vi "UI_Queue_Enqueue.vi"(8 "error in (no error)":errorcluster, 10 "UI Commands":cluster{"Cmd":string, "Value":variant}[](array[cluster]), 11 "Queue in":refnum<queue>) -> (0 "error out":errorcluster, 3 "Queue out":refnum<queue>)   [LabVIEW 2016]
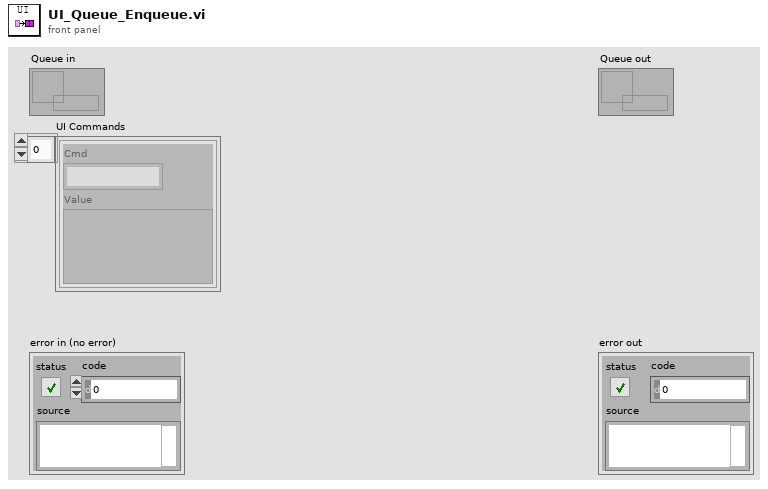
[diagram p1: front panel]
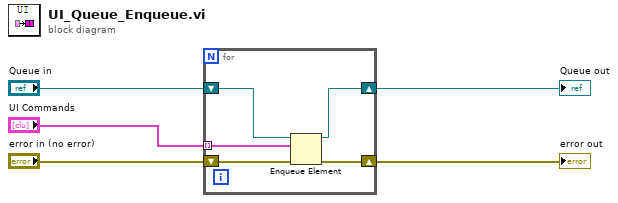
[diagram p0: block diagram]
diagram:
  n1 = for {
    shift-right: [w10] -> w5
    shift-left: "error in (no error)" -> [w9]
    shift-right: [w8] -> w3
    shift-left: "Queue in" -> [w7]
    tunnel: "UI Commands" -> [w6] mode=indexing
    n2 = Enqueue Element(queue=w7, element=w6, error in (no error)=w9) -> (queue out=w8:refnum<queue>, error out=w10:errorcluster)  [unwired: 1 in, 1 out]
  }
  "error out" <- w5
  "Queue out" <- w3
